vi "Read VISA Handle.vi"(8 "error in (no error)":errorcluster, 11 "smc100 in":refnum<class "smc100.lvclass">) -> (0 "error out":errorcluster, 2 "VISA Handle":refnum<visa-resource-name>, 3 "smc100 out":refnum<class "smc100.lvclass">)   [LabVIEW 2019, in "smc100.lvlib" / "smc100.lvclass"]
uses:
  smc100.lvclass
  smc100.lvclass/smc100.ctl
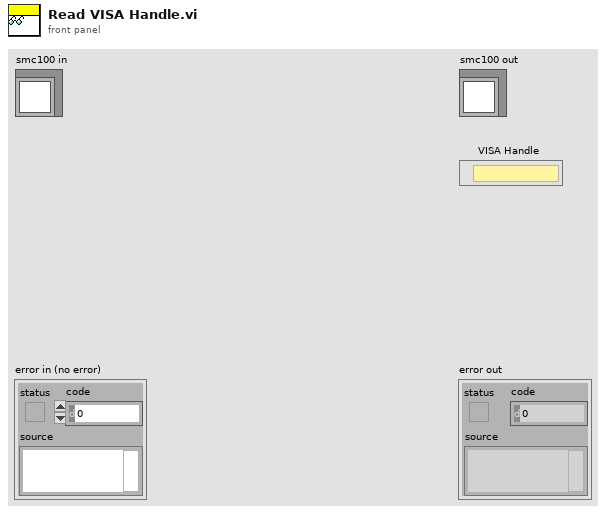
[diagram p1: front panel]
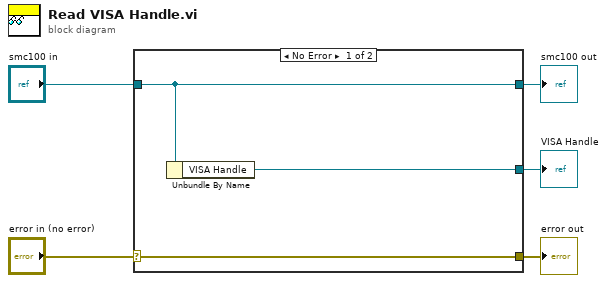
[diagram p0: block diagram]
diagram:
  n1 = case shown="No Error" "error in (no error)" {
    selector: "error in (no error)" -> [w8 w9]
    tunnel: [w8 w9] -> w4
    tunnel: [w7 w10] -> w2
    tunnel: "smc100 in" -> [w7 w10]
    tunnel: [w6 _] -> w1
    frame No Error {
      n2 = Unbundle By Name(w7) -> ("VISA Handle"=w6:refnum<visa-resource-name>)
    }
    frame Error {
    }
  }
  "error out" <- w4
  "smc100 out" <- w2
  "VISA Handle" <- w1
